vi "PIO.Read (1D DBL).vi"(8 "error in (no error)":errorcluster, 9 "count":u32, 10 "offset":u32 format="%.0x", 11 "GE 5565PIORC in":refnum<class "GE 5565PIORC Old.lvclass">) -> (0 "error out":errorcluster, 2 "values":dbl[](array[numeric]), 3 "GE 5565PIORC out":refnum<class "GE 5565PIORC Old.lvclass">)   [LabVIEW 2016, in "GE 5565PIORC Old.lvclass"]
uses:
  GE 5565PIORC Old.lvclass
  GE 5565PIORC Old.lvclass/GE 5565PIORC Old.ctl
  SubVIs/PIO.Read U32 Array.vi
  SubVIs/Byte Count to U32 Transfers.vi
  SubVIs/Change Endianness (1D U32).vi
  SubVIs/Change Endianness (U32).vi
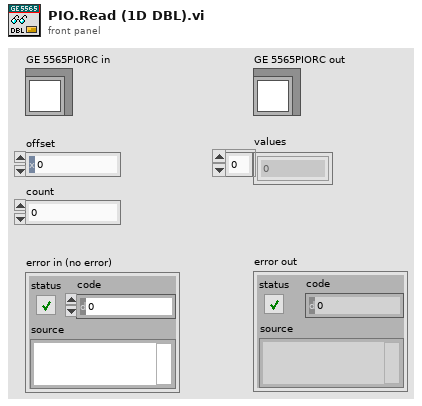
[diagram p1: front panel]
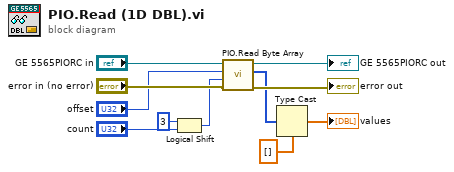
[diagram p0: block diagram]
diagram:
  n1 = Logical Shift(y=i16 3, x="count") -> (x << y=w3:u32)
  n2 = call "PIO.Read Byte Array.vi"("error in (no error)"="error in (no error)", "count"=w3, "offset"="offset", "GE 5565PIORC in"="GE 5565PIORC in") -> ("error out"=→"error out":errorcluster, "bytes read"=w1:u8[], "GE 5565PIORC out"=→"GE 5565PIORC out":refnum<class "GE 5565PIORC Old.lvclass">)  [unwired: 5 in]
  n3 = Type Cast(type=dbl[] [], x=w1) -> (*(type *) &x=→"values":dbl[])
